vi "ScanPort.vi"(4 "Command":string, 6 "Start Delay":dbl=5.0, 8 "Error In":errorcluster, 10 "Timeout":u32=250, 11 "Baud Rate":string="115200") -> (0 "Error Out":errorcluster, 1 "Found":bool, 2 "Ports Found":string[](array[string]), 3 "Port":refnum<visa-resource-name>)   [LabVIEW 2010]
uses:
  <vilib>/Instr/_visa.llb/VISA Configure Serial Port (Instr).vi
panel:
  out "read buffer":string
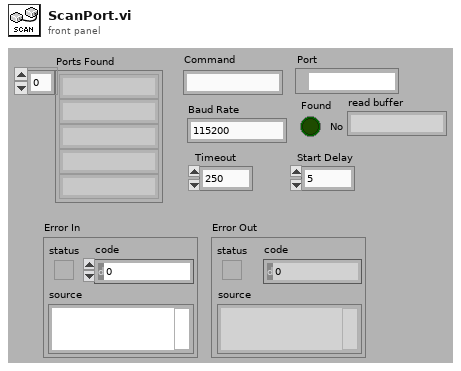
[diagram p1: front panel]
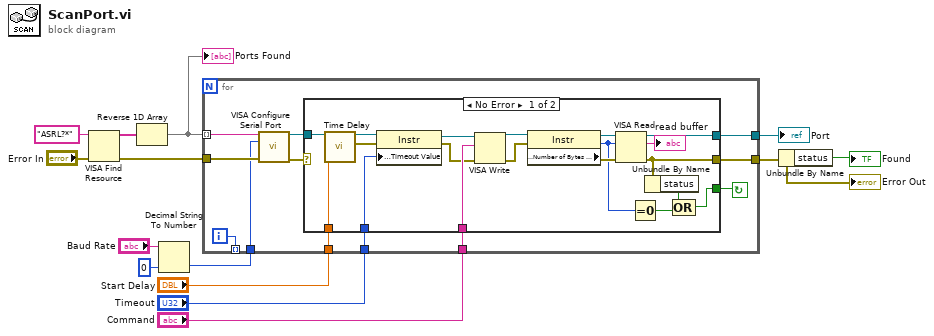
[diagram p0: block diagram]
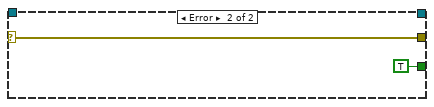
[diagram p2: hidden frame]
diagram:
  n1 = VISA Find Resource(8:"Error In", 11:"ASRL?*" ("expression (\"?*\")")) -> (0:w9:errorcluster, 3:w13:string[])  [unwired: 1 in, 1 out]
  n2 = Reverse 1D Array(array=w13) -> (reversed array=w1:string[])
  "Ports Found" <- w1
  n3 = Decimal String To Number(string="Baud Rate", default (0L)=u32 0) -> (number=w3:u32)  [unwired: 1 in, 1 out]
  n4 = for {
    tunnel: w1 -> [w26] mode=indexing
    tunnel: "Command" -> [w24]
    tunnel: "Timeout" -> [w23]
    tunnel: [w22] -> w10
    tunnel: [w16] -> w5
    tunnel: w9 -> [w21]
    tunnel: w3 -> [w20]
    tunnel: "Start Delay" -> [w19]
    tunnel: [w17] -> _ mode=indexing
    i -> [w17]
    stop <- w15 continue-if-true
    n5 = call-poly "VISA Configure Serial Port"("VISA resource name"=w26, "baud rate (9600)"=w20, "error in (no error)"=w21) -> ("VISA resource name out"=w25:refnum<visa-resource-name>, "error out"=w18:errorcluster)  [unwired: 11 in]
    n6 = case shown="No Error" w18 {
      selector: w18 -> [_ w46]
      tunnel: w25 -> [w44 _]
      tunnel: w24 -> [w43 _]
      tunnel: w23 -> [w41 _]
      tunnel: [w35 _] -> w22
      tunnel: [w32 w46] -> w16
      tunnel: w19 -> [w33 _]
      tunnel: [w28 TRUE ("status")] -> w15
      frame No Error {
        n7 = call "Time Delay"("Delay Time (s)"=w33) -> ("error out"=w34:errorcluster)  [unwired: 10 in]
        n8 = property class="Instr"(reference=w44, error in=w34, "General Settings:Timeout Value"=w41) -> (reference out=w42:refnum<visa-resource-name>, error out=w40:errorcluster)
        n9 = VISA Write(VISA resource name=w42, write buffer=w43, error in (no error)=w40) -> (VISA resource name out=w38:refnum<visa-resource-name>, error out=w39:errorcluster)  [unwired: 1 out]
        n10 = property class="Instr"(reference=w38, error in=w39) -> (reference out=w37:refnum<visa-resource-name>, error out=w36:errorcluster, "Serial Settings:Number of Bytes at Serial Port"=w29:u32)
        n11 = VISA Read(VISA resource name=w37, byte count=w29, error in (no error)=w36) -> (VISA resource name out=w35:refnum<visa-resource-name>, read buffer=→"read buffer":string, error out=w32:errorcluster)  [unwired: 1 out]
        n12 = Equal To 0?(x=w29) -> (x = 0?=w31:bool)
        n13 = Unbundle By Name(w32) -> ("status"=w30:bool)
        n14 = Compound Arithmetic op=OR(w30, w31) -> (w28:bool)
      }
      frame Error {
      }
    }
  }
  "Port" <- w10
  "Error Out" <- w5
  n15 = Unbundle By Name(w5) -> ("status"=→"Found":bool)
